vi "Teleop.vi"(10 "Match Info":T1={"Autonomous Elapsed Seconds"=0.0, "TeleOp Elapsed Seconds"=0.0, "Disabled Elapsed Seconds"=0.0, "Visited Autonomous"=FALSE, "Visited TeleOp"=FALSE, "Visited Disabled"=FALSE, "Autonomous Settings"={"Autonomous Style"=enum."Independent", "VI Refnum"=refnum}}, 11 "Call Context":T2) -> ()   [LabVIEW 2017]
doc: "This VI is called for each TeleOp packet received from the DS where the robot is not disabled. It is often used to read from the joysticks and update I/O or to update setpoints for timed control loops. It should complete and return within 20 milliseconds or it may miss DS packets."
uses:
  <vilib>/Rock Robotics/WPI/DriverStation/WPI_DriverStationDerivedRobotMode.ctl
  <vilib>/Rock Robotics/WPI/DriverStation/WPI_DriverStationMatch Info.ctl
  <vilib>/Rock Robotics/WPI/Solenoid/WPI_SolenoidValue.ctl
  <vilib>/Rock Robotics/WPI/Utilities/WPI_GetSetVariantRefNum.vi
  <vilib>/Rock Robotics/Network Tables/NT Write Boolean Array.vi
  <vilib>/Rock Robotics/Network Tables/NT Write Numeric Array.vi
  <vilib>/Rock Robotics/Network Tables/NT Read Boolean.vi
  <vilib>/Rock Robotics/Network Tables/NT Read Number.vi
  <vilib>/Rock Robotics/WPI/ThirdParty/Phoenix-LabVIEW/Motor Controller/Get/CTRE_Phoenix_MotorController_GetOutputCurrent_Enhanced.vi
  <vilib>/Rock Robotics/WPI/ThirdParty/Phoenix-LabVIEW/Motor Controller/Get/CTRE_Phoenix_MotorController_GetVoltage.vi
  <vilib>/Rock Robotics/WPI/ThirdParty/Phoenix-LabVIEW/Motor Controller/Get/CTRE_Phoenix_MotorController_GetSelectedSensorData.vi
  <vilib>/Rock Robotics/WPI/Solenoid/WPI_SolenoidSetEnum.vi
panel:
  out "Right Current":dbl
  out "Left Current":dbl
  out "Ultra Sonic Distance Inches":dbl
  out "Right Voltage":dbl
  out "Left Voltage":dbl
  out "Right Encoder Rotations":dbl format="%.2f"
  out "Left Encoder Rotations":dbl format="%.2f"
  out "Right Encoder Inches":dbl format="%.2f"
  out "Left Encoder Inchers":dbl format="%.2f"
  out "Right Encoder":i32
  out "Left Encoder":i32
  out "Sample Slider 0":dbl(slide) scale=0.0..5.0
  out "Sample Boolean 1":bool
  out "Sample Boolean 0":bool
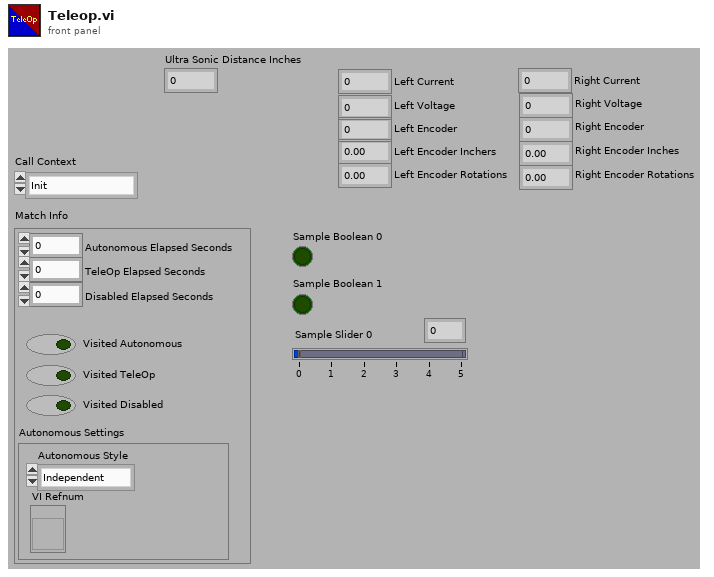
[diagram p1: front panel]
types:
  T1 = typedef "WPI_DriverStationMatch Info.ctl" = cluster{"Autonomous Elapsed Seconds":dbl, "TeleOp Elapsed Seconds":dbl, "Disabled Elapsed Seconds":dbl, "Visited Autonomous":bool, "Visited TeleOp":bool, "Visited Disabled":bool, "Autonomous Settings":cluster{"Autonomous Style":enum16{"Iterative", "Independent"}, "VI Refnum":refnum<vi>}}
  T2 = typedef "WPI_DriverStationDerivedRobotMode.ctl" = enum16{"Init", "Execute", "Stop"}
  T3 = typedef "WPI_SolenoidValue.ctl" = enum16{"Off", "On", "Forward", "Reverse"}
  T4 = typedef "WPI_JoystickDevRef.ctl" = cluster{"Device":T5}
  T5 = typedef "WPI_JoystickDeviceEnum.ctl" = enum16{"USB 0", "USB 1", "USB 2", "USB 3", "USB 4", "USB 5"}
  T6 = cluster{"Buttons[0]":bool, "Buttons[1]":bool, "Buttons[2]":bool, "Buttons[3]":bool, "Buttons[4]":bool, "Buttons[5]":bool, "Buttons[6]":bool, "Buttons[7]":bool, "Buttons[8]":bool}
  T7 = typedef "WPI_RobotDriveDevRef.ctl" = cluster{"DevStatus":errorcluster, "Motors[]":T8[], "Square Inputs":bool, "Max Output":dbl}
  T8 = typedef "WPI_MotorControlDeviceRef.ctl" = cluster{"DeviceStatus":errorcluster, "Type":T9, "PWM":cluster{"PWM Channel":T10, "DeadBand":T11}, "CAN":cluster{"Device Number":u8, "SetOutput VI Ref":variant, "GetOutput VI Ref":variant, "Enable VI Ref":variant, "Disable VI Ref":variant, "Data":variant}, "Invert":bool, "DIO PWM":cluster{"PWM \"Enable\" Channel":T10, "DIOChannel":T12, "PWM Rate":dbl}}
  T9 = typedef "WPI_MotorControlType.ctl" = enum16{"PWM", "CAN", "DIO PWM"}
  T10 = typedef "FPGA_DIOPWMChannel.ctl" = enum8{"PWM 0", "PWM 1", "PWM 2", "PWM 3", "PWM 4", "PWM 5", "PWM 6", "PWM 7", "PWM 8", "PWM 9", "PWM MXP 0", "PWM MXP 1", "PWM MXP 2", "PWM MXP 3", "PWM MXP 4", "PWM MXP 5", "PWM MXP 6", "PWM MXP 7", "PWM MXP 8", "PWM MXP 9", "Invalid"}
  T11 = typedef "WPI_PWMDeadband.ctl" = cluster{"Name":string, "maxPositivePwm":i32, "minPositivePwm":i32, "centerPwm":i32, "maxNegativePwm":i32, "minNegativePwm":i32, "angularRange":u16}
  T12 = typedef "FPGA_DIOChannel.ctl" = enum8{"DIO 0", "DIO 1", "DIO 2", "DIO 3", "DIO 4", "DIO 5", "DIO 6", "DIO 7", "DIO 8", "DIO 9", "DIO MXP 0", "DIO MXP 1", "DIO MXP 2", "DIO MXP 3", "DIO MXP 4", "DIO MXP 5", "DIO MXP 6", "DIO MXP 7", "DIO MXP 8", "DIO MXP 9", "DIO MXP 10", "DIO MXP 11", "DIO MXP 12", "DIO MXP 13", "DIO MXP 14", "DIO MXP 15", "SPI Port CS1", "SPI Port CS2", "SPI Port CS3", "SPI Port MISO", "SPI Port MOSI", "Invalid"}
  T13 = cluster{"Axes[0]":dbl, "Axes[1]":dbl, "Axes[2]":dbl, "Axes[3]":dbl, "Axes[4]":dbl, "Axes[5]":dbl, "Axes[6]":dbl, "Axes[7]":dbl, "Axes[8]":dbl}
  T14 = typedef "WPI_AnalogChannelDevRef.ctl" = cluster{"DevStatus":errorcluster, "Analog Channel":T15}
  T15 = typedef "FPGA_AIChannel.ctl" = enum8{"AI 0", "AI 1", "AI 2", "AI 3", "AI MXP 0", "AI MXP 1", "AI MXP 2", "AI MXP 3", "Invalid"}
  T16 = typedef "WPI_SolenoidDevRef.ctl" = cluster{"DevStatus":errorcluster, "Pneumatics Control Module":u8, "Forward Solenoid Channel":T17, "Reverse Solenoid Channel":T17}
  T17 = typedef "WPI_SolenoidChannel.ctl" = enum8{"Solenoid 0", "Solenoid 1", "Solenoid 2", "Solenoid 3", "Solenoid 4", "Solenoid 5", "Solenoid 6", "Solenoid 7", "Invalid"}
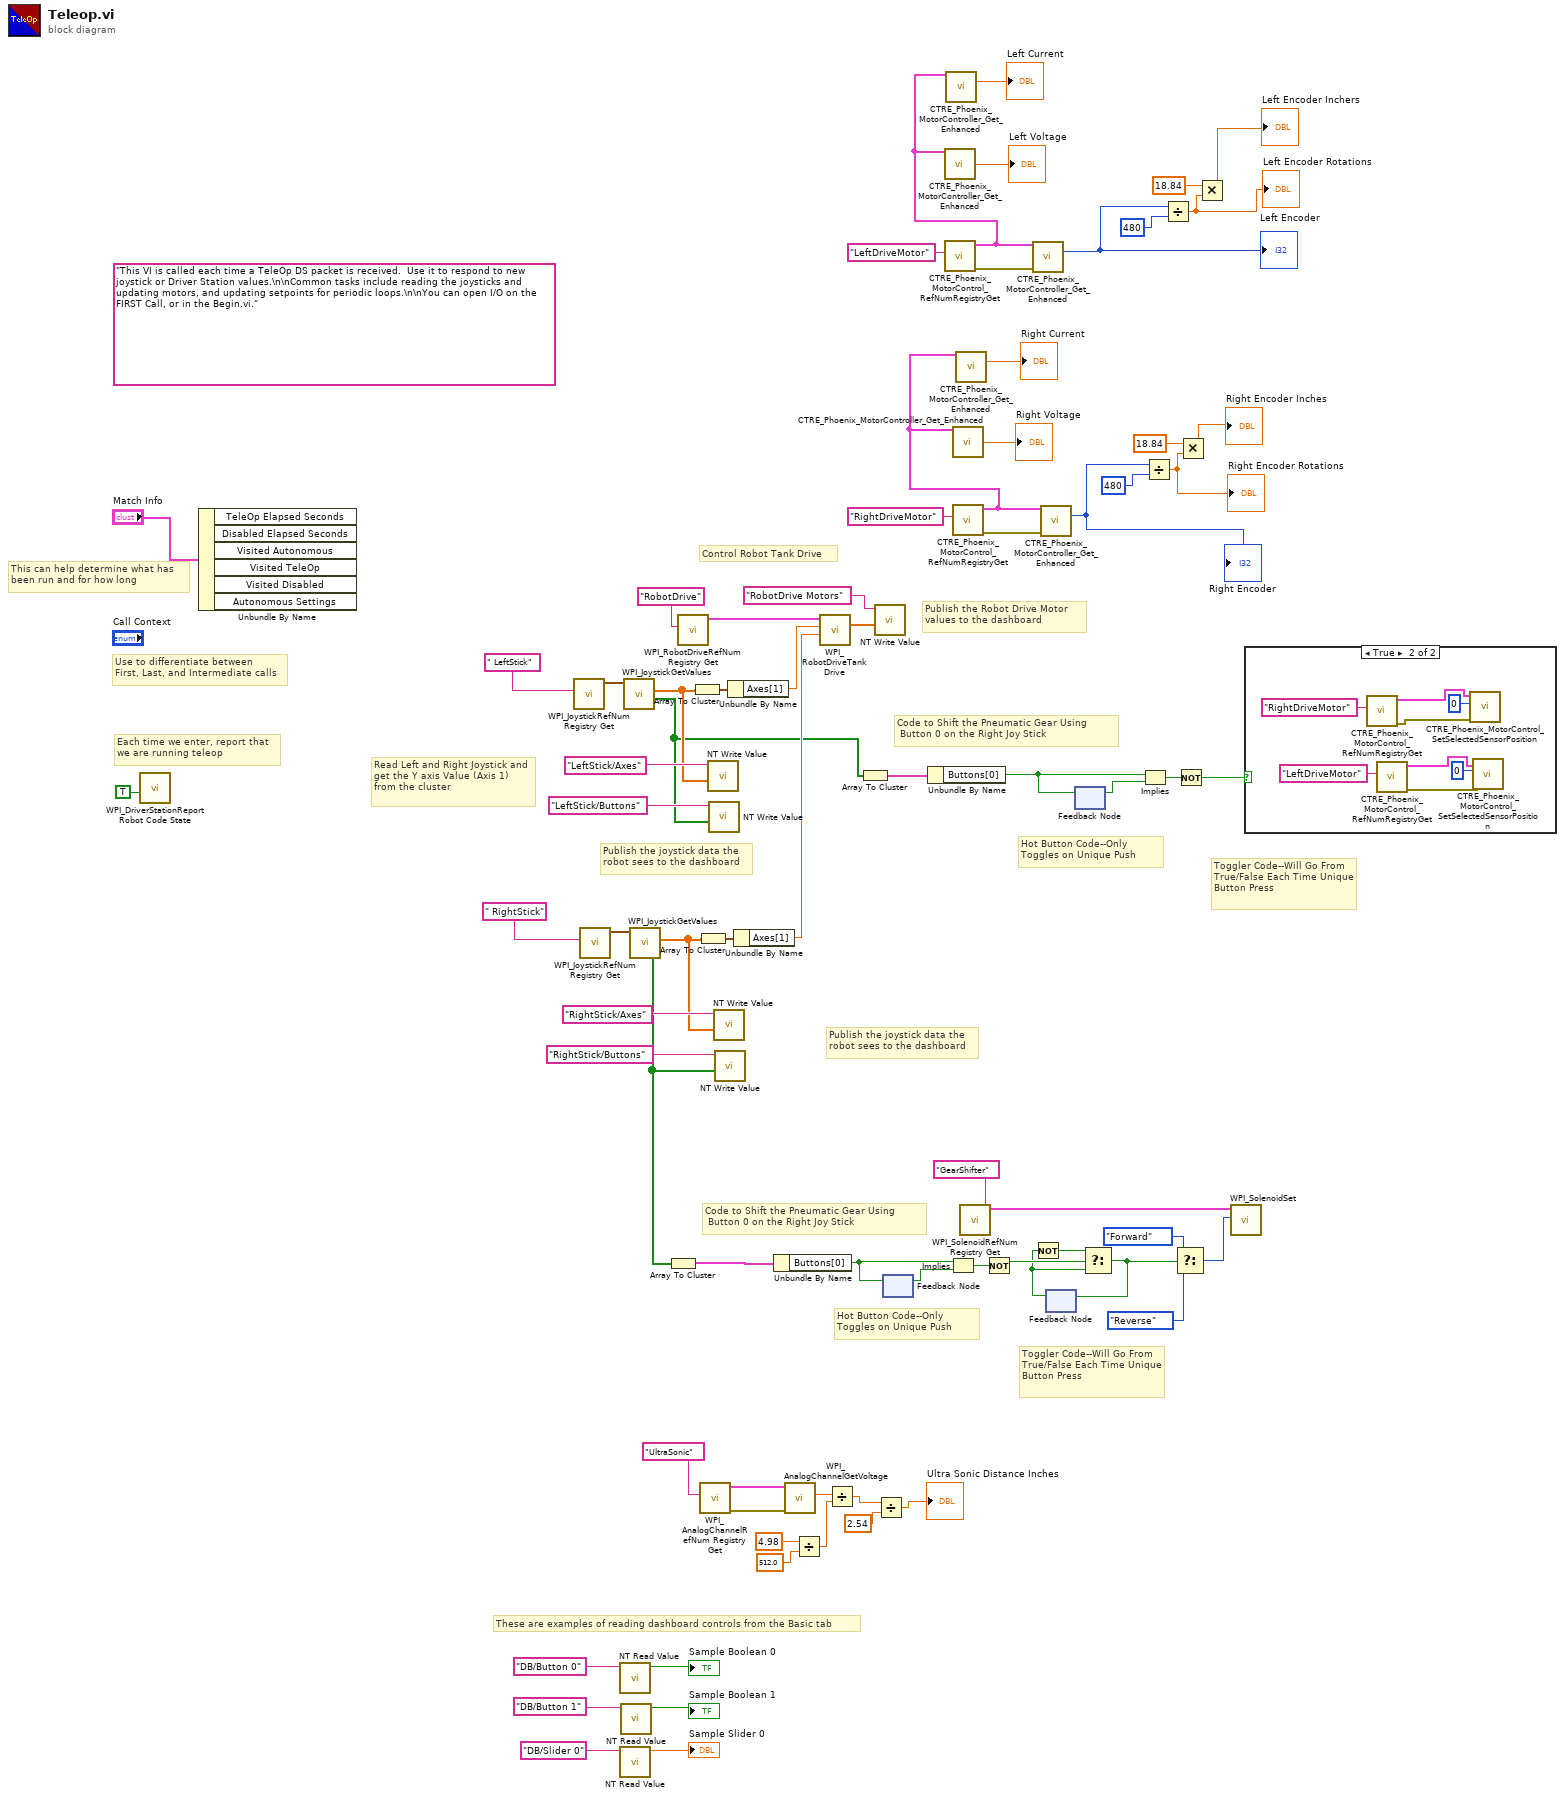
[diagram p0: block diagram]
diagram:
  (unwired) "This VI is called each time a TeleOp DS packet is received.  Use it to respond to new joystick or Driver Station values.\n\nCommon tasks include reading the joysticks and updating motors, and updating setpoints for periodic loops.\n\nYou can open I/O on the FIRST Call, or in the Begin.vi."
  # "Toggler Code--Will Go From True/False Each Time Unique Button Press"
  # "Hot Button Code--Only \nToggles on Unique Push"
  # "Code to Shift the Pneumatic Gear Using\n Button 0 on the Right Joy Stick"
  # "Control Robot Tank Drive"
  # "Toggler Code--Will Go From True/False Each Time Unique Button Press"
  # "Hot Button Code--Only \nToggles on Unique Push"
  # "Code to Shift the Pneumatic Gear Using\n Button 0 on the Right Joy Stick"
  # "Publish the joystick data the\nrobot sees to the dashboard"
  # "These are examples of reading dashboard controls from the Basic tab"
  # "Publish the Robot Drive Motor\nvalues to the dashboard"
  # "Publish the joystick data the\nrobot sees to the dashboard"
  # "Each time we enter, report that\nwe are running teleop"
  # "Use to differentiate between\nFirst, Last, and Intermediate calls"
  # "This can help determine what has\nbeen run and for how long"
  # "Read Left and Right Joystick and get the Y axis Value (Axis 1) from the cluster"
  n1 = call <vilib>:"WPI_DriverStationReport Robot Code State.vi"("TeleOp"=TRUE ("Autonomous")) -> ()  [unwired: 10 in, 1 out]
  n2 = Unbundle By Name("Match Info") -> ()  [unwired: 6 out]
  n3 = call <vilib>:"WPI_JoystickRefNum Registry Get.vi"("refnum name"=" LeftStick") -> ("JoystickDevRef"=w72:T4)  [unwired: 1 in, 9 out]
  n4 = call <vilib>:"WPI_JoystickRefNum Registry Get.vi"("refnum name"=" RightStick") -> ("JoystickDevRef"=w56:T4)  [unwired: 1 in, 9 out]
  n5 = call-poly <vilib>:"NT Read Value.vi"("Name"="DB/Button 0" ("refnum name")) -> ("Boolean"=→"Sample Boolean 0":bool)  [unwired: 9 in, 1 out]
  n6 = call-poly <vilib>:"NT Read Value.vi"("Name"="DB/Slider 0" ("refnum name")) -> ("Numeric"=→"Sample Slider 0":dbl)  [unwired: 9 in, 1 out]
  n7 = call-poly <vilib>:"NT Read Value.vi"("Name"="DB/Button 1" ("refnum name")) -> ("Boolean"=→"Sample Boolean 1":bool)  [unwired: 9 in, 1 out]
  n8 = call <vilib>:"WPI_JoystickGetValues.vi"("JoystickDevRef"=w72) -> ("Buttons"=w5:bool[], "Axes"=w60:dbl[])  [unwired: 6 in, 3 out]
  n9 = call <vilib>:"WPI_JoystickGetValues.vi"("JoystickDevRef"=w56) -> ("Buttons"=w38:bool[], "Axes"=w53:dbl[])  [unwired: 6 in, 3 out]
  n10 = Array To Cluster(array=w38) -> (cluster=w49:T6)
  n11 = call <vilib>:"WPI_RobotDriveRefNum Registry Get.vi"("refnum name"="RobotDrive") -> ("RobotDriveDevRef"=w74:T7)  [unwired: 1 in, 9 out]
  n12 = Array To Cluster(array=w60) -> (cluster=w59:T13)
  n13 = Array To Cluster(array=w53) -> (cluster=w52:T13)
  n14 = call <vilib>:"WPI_AnalogChannelRefNum Registry Get.vi"("refnum name"="UltraSonic") -> ("error out"=w19:errorcluster, "AIDeviceRef"=w20:T14)  [unwired: 9 in]
  n15 = call-poly <vilib>:"NT Write Value.vi"("Numeric Array"=w60, "Name"="LeftStick/Axes") -> ()  [unwired: 9 in, 1 out]
  n16 = call-poly <vilib>:"NT Write Value.vi"("Boolean Array"=w5, "Name"="LeftStick/Buttons") -> ()  [unwired: 9 in, 1 out]
  n17 = call-poly <vilib>:"NT Write Value.vi"("Numeric Array"=w53, "Name"="RightStick/Axes") -> ()  [unwired: 9 in, 1 out]
  n18 = call-poly <vilib>:"NT Write Value.vi"("Boolean Array"=w38, "Name"="RightStick/Buttons") -> ()  [unwired: 9 in, 1 out]
  n19 = Unbundle By Name(w59) -> ("Axes[1]"=w58:dbl)
  n20 = Unbundle By Name(w52) -> ("Axes[1]"=w51:dbl)
  n21 = Unbundle By Name(w49) -> ("Buttons[0]"=w44:bool)
  n22 = call <vilib>:"WPI_AnalogChannelGetVoltage.vi"("error in (no error)"=w19, "AIDeviceRef"=w20) -> ("Voltage"=w15:dbl)  [unwired: 7 in, 2 out]
  n23 = Divide(x=4.98, y=512.0) -> (x/y=w14:dbl)
  n24 = call <vilib>:"WPI_RobotDriveTankDrive.vi"("Right axis value"=w51, "Left axis value"=w58, "RobotDriveDevRef"=w74) -> ("Motor Values"=w62:dbl[])  [unwired: 6 in, 2 out]
  n25 = Divide(x=w15, y=w14) -> (x/y=w9:dbl)
  n26 = Array To Cluster(array=w5) -> (cluster=w4:T6)
  n27 = call-poly <vilib>:"NT Write Value.vi"("Numeric Array"=w62, "Name"="RobotDrive Motors") -> ()  [unwired: 9 in, 1 out]
  n28 = Divide(x=w9, y=2.54) -> (x/y=→"Ultra Sonic Distance Inches":dbl)
  n29 = feedback #1() -> (w37:bool)  [unwired: 1 in]
  n30 = feedback-in #1(w44) -> ()
  n31 = Unbundle By Name(w4) -> ("Buttons[0]"=w3:bool)
  n32 = call <vilib>:"CTRE_Phoenix_MotorControl_RefNumRegistryGet.vi"("refnum name"="LeftDriveMotor") -> ("error out"=w35:errorcluster, "PhoenixMotorControlDevRef"=w13:T8)  [unwired: 9 in]
  n33 = call-poly <vilib>:"CTRE_Phoenix_MotorController_Get_Enhanced.vi"("PhoenixMotorControlDevRef"=w13) -> ("Output Voltage"=→"Left Voltage":dbl)  [unwired: 10 in, 4 out]
  n34 = call-poly <vilib>:"CTRE_Phoenix_MotorController_Get_Enhanced.vi"("PhoenixMotorControlDevRef"=w13) -> ("Output Current"=→"Left Current":dbl)  [unwired: 12 in, 2 out]
  n35 = Implies(1:w37, 2:w44) -> (0:w48:bool)
  n36 = call <vilib>:"CTRE_Phoenix_MotorControl_RefNumRegistryGet.vi"("refnum name"="RightDriveMotor") -> ("error out"=w33:errorcluster, "PhoenixMotorControlDevRef"=w10:T8)  [unwired: 9 in]
  n37 = call-poly <vilib>:"CTRE_Phoenix_MotorController_Get_Enhanced.vi"("PhoenixMotorControlDevRef"=w10) -> ("Output Voltage"=→"Right Voltage":dbl)  [unwired: 10 in, 4 out]
  n38 = call-poly <vilib>:"CTRE_Phoenix_MotorController_Get_Enhanced.vi"("PhoenixMotorControlDevRef"=w10) -> ("Output Current"=→"Right Current":dbl)  [unwired: 12 in, 2 out]
  n39 = call <vilib>:"WPI_SolenoidRefNum Registry Get.vi"("refnum name"="GearShifter") -> ("SolenoidDevRef"=w43:T16)  [unwired: 9 in, 1 out]
  n40 = Not(x=w48) -> (.not. x?=w47:bool)
  n41 = call-poly <vilib>:"CTRE_Phoenix_MotorController_Get_Enhanced.vi"("PhoenixMotorControlDevRef"=w13, "error in"=w35) -> ("Position (Raw Sensor Units)"=w32:i32)  [unwired: 10 in, 3 out]
  "Left Encoder" <- w32
  n42 = call-poly <vilib>:"CTRE_Phoenix_MotorController_Get_Enhanced.vi"("PhoenixMotorControlDevRef"=w10, "error in"=w33) -> ("Position (Raw Sensor Units)"=w25:i32)  [unwired: 10 in, 3 out]
  "Right Encoder" <- w25
  n43 = feedback #2() -> (w45:bool)  [unwired: 1 in]
  n44 = Not(x=w45) -> (.not. x?=w46:bool)
  n45 = feedback #3() -> (w2:bool)  [unwired: 1 in]
  n46 = feedback-in #3(w3) -> ()
  n47 = Select(t=w46, s=w47, f=w45) -> (s? t:f=w42:bool)
  n48 = feedback-in #2(w42) -> ()
  n49 = Implies(1:w2, 2:w3) -> (0:w6:bool)
  n50 = Divide(x=w25, y=480) -> (x/y=w23:dbl)
  "Right Encoder Rotations" <- w23
  n51 = Divide(x=w32, y=480) -> (x/y=w24:dbl)
  "Left Encoder Rotations" <- w24
  n52 = Select(t=WPI_SolenoidValue."Forward" ("Value"), s=w42, f=WPI_SolenoidValue."Reverse" ("Value")) -> (s? t:f=w39:T3)
  n53 = Not(x=w6) -> (.not. x?=w1:bool)
  n54 = Multiply(x=18.84, y=w23) -> (x*y=→"Right Encoder Inches":dbl)
  n55 = Multiply(x=18.84, y=w24) -> (x*y=→"Left Encoder Inchers":dbl)
  n56 = call-poly <vilib>:"WPI_SolenoidSet.vi"("Value"=w39, "SolenoidDevRef"=w43) -> ()  [unwired: 8 in, 2 out]
  n57 = case shown="True" w1 {
    frame False {
    }
    frame True {
      n58 = call <vilib>:"CTRE_Phoenix_MotorControl_RefNumRegistryGet.vi"("refnum name"="RightDriveMotor") -> ("error out"=w80:errorcluster, "PhoenixMotorControlDevRef"=w81:T8)  [unwired: 9 in]
      n59 = call <vilib>:"CTRE_Phoenix_MotorControl_RefNumRegistryGet.vi"("refnum name"="LeftDriveMotor") -> ("error out"=w77:errorcluster, "PhoenixMotorControlDevRef"=w78:T8)  [unwired: 9 in]
      n60 = call <vilib>:"CTRE_Phoenix_MotorControl_SetSelectedSensorPosition.vi"("error in (no error)"=w80, "New Sensor Position"=0, "PhoenixMotorControlDevRef"=w81) -> ()  [unwired: 7 in, 2 out]
      n61 = call <vilib>:"CTRE_Phoenix_MotorControl_SetSelectedSensorPosition.vi"("error in (no error)"=w77, "New Sensor Position"=0, "PhoenixMotorControlDevRef"=w78) -> ()  [unwired: 7 in, 2 out]
    }
  }
